vi "Untitled 21.vi"() -> ()   [LabVIEW 2015]
uses:
  Sequencer/Sequencer/Daq Channel Info.ctl
  <resource>/objmgr/daqmx.rc
  Sequencer/Sequencer/Sequencer.lvclass
panel:
  out "Used DAQChannels":tag[](array[tag])
  out "output array":tag[](array[tag])
  out "output cluster":T1
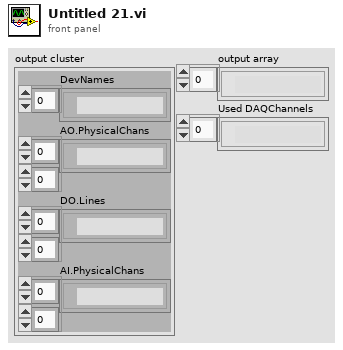
[diagram p1: front panel]
types:
  T1 = typedef "Sequencer.lvlib/Sequencer.lvclass/Daq Channel Info.ctl" = cluster{"DevNames":tag[], "AO.PhysicalChans":tag[][], "DO.Lines":tag[][], "AI.PhysicalChans":tag[][]}
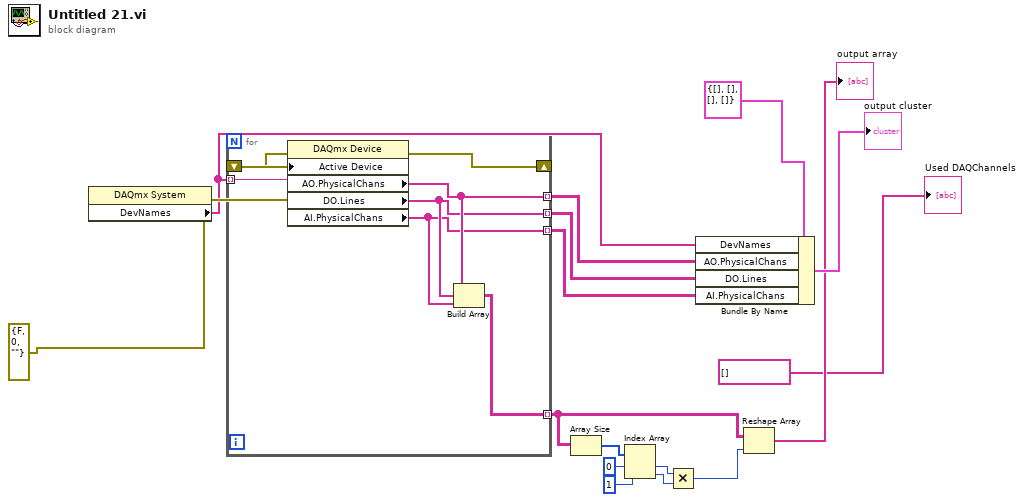
[diagram p0: block diagram]
diagram:
  n1 = property class="DAQmx System"(error in=errorcluster {"status"=FALSE, "code"=0, "source"=""} ("error in (no error)")) -> (error out=w17:errorcluster, "DevNames"=w16:tag[])  [unwired: 1 in, 1 out]
  n2 = for {
    tunnel: w16 -> [w24] mode=indexing
    tunnel: [w21] -> w13 mode=indexing
    tunnel: [w20] -> w14 mode=indexing
    tunnel: [w19] -> w15 mode=indexing
    shift-right: [w22] -> _
    shift-left: w17 -> [w23]
    tunnel: [w18] -> w7 mode=indexing
    n3 = property class="DAQmx Device"(error in=w23, "Active Device"=w24) -> (error out=w22:errorcluster, "AO.PhysicalChans"=w21:tag[], "DO.Lines"=w20:tag[], "AI.PhysicalChans"=w19:tag[])  [unwired: 1 in, 1 out]
    n4 = Build Array(w21, w20, w19) -> (w18:tag[][])
  }
  n5 = Array Size(array=w7) -> (size(s)=w12:i32[])
  n6 = Index Array(array=w12, index #1=0 ("index"), index #2=1 ("index")) -> (element #1=w9:i32, element #2=w8:i32)
  n7 = Multiply(x=w9, y=w8) -> (x*y=w6:i32)
  n8 = Bundle By Name(cluster=T1 {"DevNames"=[], "AO.PhysicalChans"=[], "DO.Lines"=[], "AI.PhysicalChans"=[]} ("Daq Channel Info"), "DevNames"=w16, "AO.PhysicalChans"=w13, "DO.Lines"=w14, "AI.PhysicalChans"=w15) -> (→"output cluster":T1)
  n9 = Reshape Array(w7, w6) -> (→"output array":tag[])
  "Used DAQChannels" <- tag[] [] ("Used DAQChannels")
